vi "HighScore.vi"(8 "error in":errorcluster, 11 "score in":i32) -> (0 "error out":errorcluster, 3 "hallOfFame out":cluster{"score":i32, "name":string}[](array[cluster]))   [LabVIEW 2010, in "Labricks.lvlib" / "Game.lvclass"]
uses:
  Game.lvclass
  <vilib>/Utility/xml.llb/Read From XML File(string).vi
  <vilib>/Utility/xml.llb/Write to XML File(string).vi
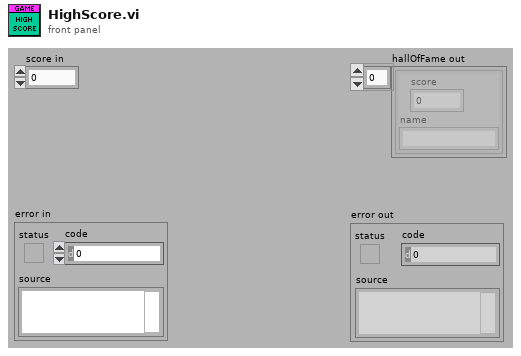
[diagram p1: front panel]
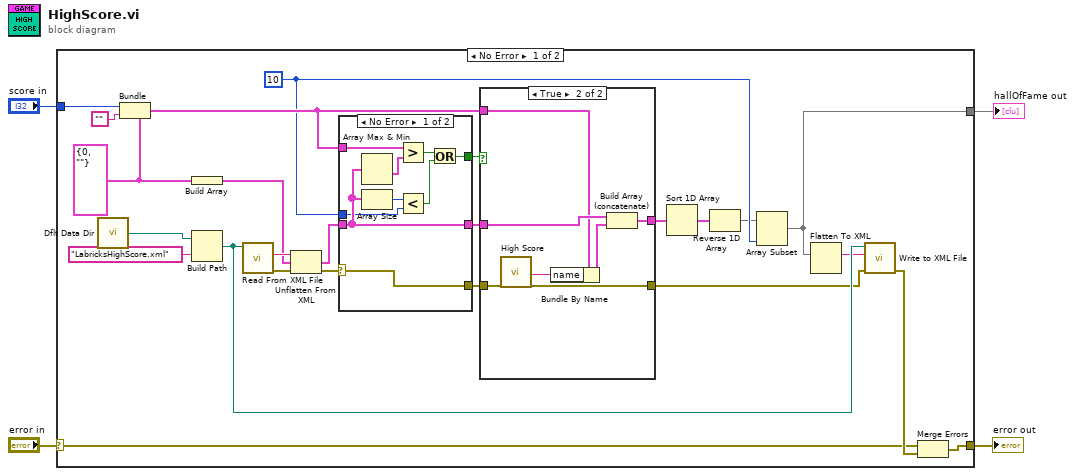
[diagram p0: block diagram]
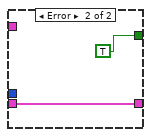
[diagram p3: hidden frame]
diagram:
  n1 = case shown="No Error" "error in" {
    selector: "error in" -> [w24 w50]
    tunnel: [w25 w50] -> w3
    tunnel: "score in" -> [w20 _]
    tunnel: [w8 _] -> w1
    frame No Error {
      w9 = 10 ("y")
      w17 = cluster{"score":i32, "name":string} {"score"=0, "name"=""}
      n2 = call <vilib>:"Dflt Data Dir.vi"() -> ("App:Default Data Directory"=w29:path)
      n3 = Bundle(cluster=w17, "score"=w20, "name"="") -> (w12:cluster{"score":i32, "name":string})
      n4 = Build Array(w17) -> (w16:cluster{"score":i32, "name":string}[])
      n5 = Build Path(base path=w29, name or relative path="LabricksHighScore.xml") -> (appended path=w27:path)
      n6 = call-poly <vilib>:"Read From XML File.vi"("XML File Path"=w27) -> ("error out"=w22:errorcluster, "XML Elements"=w21:string)  [unwired: 8 in, 1 out]
      n7 = Unflatten From XML(xml string=w21, type=w16, error in (no error)=w22) -> (value=w18:cluster{"score":i32, "name":string}[], error out=w23:errorcluster)
      n8 = case shown="No Error" w23 {
        selector: w23 -> [w46 _]
        tunnel: [w43 w49] -> w11
        tunnel: w18 -> [w43 w49]
        tunnel: w12 -> [w47 _]
        tunnel: [w46 _] -> w13
        tunnel: [w44 TRUE] -> w14
        tunnel: w9 -> [w41 _]
        frame No Error {
          n9 = Array Max & Min(array=w43) -> (min value=w39:cluster{"score":i32, "name":string})  [unwired: 3 out]
          n10 = Array Size(array=w43) -> (size(s)=w42:i32)
          n11 = Greater?(x=w47, y=w39) -> (0:w45:bool)
          n12 = Less?(x=w42, y=w41) -> (x < y?=w40:bool)
          n13 = Or(x=w45, y=w40) -> (x .or. y?=w44:bool)
        }
        frame Error {
        }
      }
      n14 = case shown="True" w14 {
        tunnel: w13 -> [w30 w38]
        tunnel: w11 -> [w31 w37]
        tunnel: [w31 w36] -> w7
        tunnel: [w30 w34] -> w10
        tunnel: w12 -> [_ w33]
        frame False {
        }
        frame True {
          n15 = call "High Score"("error in (no error)"=w38) -> ("Name"=w35:string, "error out"=w34:errorcluster)  [unwired: 16 in, 1 out]
          n16 = Bundle By Name(cluster=w33, "name"=w35) -> (w32:cluster{"score":i32, "name":string})
          n17 = Build Array (concatenate)(w37, w32) -> (w36:cluster{"score":i32, "name":string}[])
        }
      }
      n18 = Sort 1D Array(array=w7) -> (sorted array=w6:cluster{"score":i32, "name":string}[])
      n19 = Reverse 1D Array(array=w6) -> (reversed array=w5:cluster{"score":i32, "name":string}[])
      n20 = Array Subset(array=w5, length=w9) -> (w8:cluster{"score":i32, "name":string}[])  [unwired: 1 in]
      n21 = Flatten To XML(anything=w8) -> (xml string=w15:string)
      n22 = call-poly <vilib>:"Write to XML File.vi"("error in (no error)"=w10, "XML Input"=w15, "XML File Path"=w27) -> ("error out"=w26:errorcluster)  [unwired: 6 in, 2 out]
      n23 = Merge Errors(w24, w26) -> (w25:errorcluster)
    }
    frame Error {
    }
  }
  "error out" <- w3
  "hallOfFame out" <- w1
